vi "Selected Tool holder.vi"(1 "Action(GET)":enum16{"GET", "SET"}(ring), 7 "Tool in":T1, 11 "error in (no error)":errorcluster) -> (8 "Tool out":T1, 15 "error out":errorcluster)   [LabVIEW 2011]
uses:
  List of tools.ctl
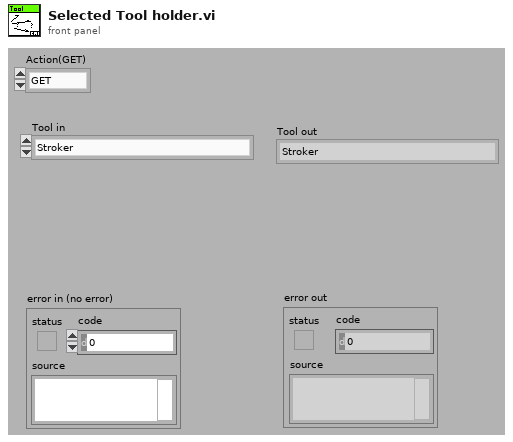
[diagram p1: front panel]
types:
  T1 = typedef "List of tools.ctl" = enum16{"Stroker", "Driller", "Tractor"}
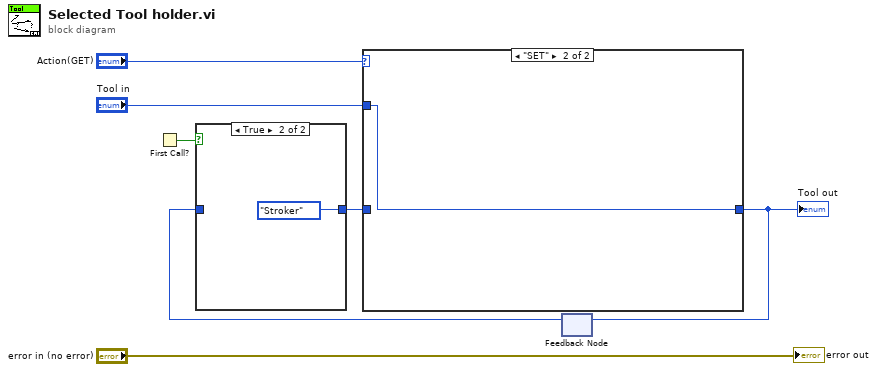
[diagram p0: block diagram]
diagram:
  n1 = First Call?() -> (First Call?: T/F=w4:bool)
  n2 = feedback #1() -> (w5:T1)  [unwired: 1 in]
  n3 = case shown="True" w4 {
    tunnel: w5 -> [w8 _]
    tunnel: [w8 List_of_tools."Stroker" ("Tool")] -> w2
    frame False {
    }
    frame True {
    }
  }
  n4 = case shown="\"SET\"" "Action(GET)" {
    tunnel: [w10 w11] -> w3
    tunnel: w2 -> [w10 _]
    tunnel: "Tool in" -> [_ w11]
    frame "GET", Default {
    }
    frame "SET" {
    }
  }
  "Tool out" <- w3
  n5 = feedback-in #1(w3) -> ()
  "error out" <- "error in (no error)"
